vi "Write GPIO Bank.vi"(0 "fpga interface in":refnum<k20>, 5 "gpio bank select":T1, 7 "gpio bank output":T2, 9 "gpio bank output enable":T2={"GPIO 0"=TRUE, "GPIO 1"=TRUE, "GPIO 2"=TRUE, "GPIO 3"=TRUE, "GPIO 4"=TRUE, "GPIO 5"=TRUE, "GPIO 6"=TRUE, "GPIO 7"=TRUE, "GPIO 8"=TRUE, "GPIO 9"=TRUE, "GPIO 10"=TRUE}, 11 "error in (no error)":errorcluster) -> (4 "fpga interface out":refnum<k20>, 15 "error out":errorcluster)   [LabVIEW 2023, in "GettingStarted_Common_148X_Host.lvlib"]
uses:
  GettingStarted_Common_148X_Host.lvlib
  <instrlib>/FlexRIO/CSI-2/v2/FPGA/Types/GPIO Bank.ctl
  FPGA/Common/Types/SerDes Identifier.ctl
  Types/148x_Common_FPGA_Reference.ctl
  <vilib>/rvi/errors/niLvFpgaAdjustHostInterfaceError.vi
  <vilib>/rvi/interface/nirviReadWriteControl/nirviReadWriteControl.xnode
  FPGA/Common/GettingStarted_Common_148X_FPGA.lvlib
  NiFpgaLv.dll
  <vilib>/rvi/interface/Simulation/niFpgaSimulationCallBeginRW.vi
  <instrlib>/FlexRIO/CSI-2/v2/FPGA/NI CSI-2 API FPGA v2.lvlib
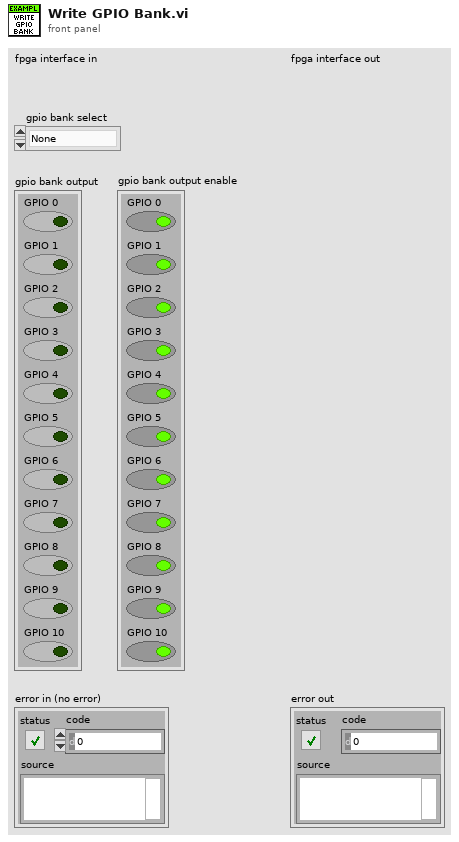
[diagram p1: front panel]
types:
  T1 = typedef "GettingStarted_Common_148X_FPGA.lvlib/SerDes Identifier.ctl" = enum8{"None", "SI 0 Deserializer", "SI 1 Deserializer", "SI 2 Deserializer", "SI 3 Deserializer", "SI 4 Deserializer", "SI 5 Deserializer", "SI 6 Deserializer", "SI 7 Deserializer", "SO 0 Serializer", "SO 1 Serializer", "SO 2 Serializer", "SO 3 Serializer", "SO 4 Serializer", "SO 5 Serializer", "SO 6 Serializer", "SO 7 Serializer", "SI 0 SI 1 Deserializer", "SI 2 SI 3 Deserializer", "SI 4 SI 5 Deserializer", "SI 6 SI 7 Deserializer"}
  T2 = typedef "NI CSI-2 API FPGA v2.lvlib/GPIO Bank.ctl" = cluster{"GPIO 0":bool, "GPIO 1":bool, "GPIO 2":bool, "GPIO 3":bool, "GPIO 4":bool, "GPIO 5":bool, "GPIO 6":bool, "GPIO 7":bool, "GPIO 8":bool, "GPIO 9":bool, "GPIO 10":bool}
  T3 = typedef "GettingStarted_Common_148X_Host.lvlib/148x_Common_FPGA_Reference.ctl" = refnum<k20>
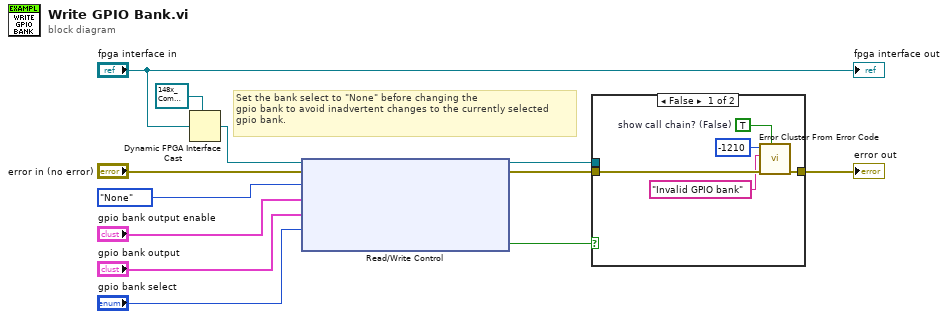
[diagram p0: block diagram]
diagram:
  # "Set the bank select to \"None\" before changing the \ngpio bank to avoid inadvertent changes to the currently selected\ngpio bank."
  n1 = Dynamic FPGA Interface Cast(Session In=T3 refnum ("FPGA VI Reference Out"), Type="fpga interface in") -> (Session Out=w11:T3)
  n2 = xnode "Read/Write Control"("FPGA VI Reference In"=w11, "error in"="error in (no error)", "gpio bank output select"=SerDes_Identifier."None", "gpio bank output enable"="gpio bank output enable", "gpio bank output"="gpio bank output", "gpio bank output select"="gpio bank select") -> ("FPGA VI Reference Out"=w7:T3, "error out"=w8:errorcluster, "serdes gpio bank output select valid"=w3:bool)
  n3 = case shown="False" w3 {
    tunnel: w8 -> [w17 w18]
    tunnel: [w16 w18] -> w6
    tunnel: w7 -> [_ _]
    frame False {
      w13 = TRUE  # show call chain? (False)
      n4 = call <vilib>:"Error Cluster From Error Code.vi"("show call chain? (False)"=w13, "error in (no error)"=w17, "error message (\"\")"="Invalid GPIO bank" ("error message (\"\")"), "error code (0)"=-1210) -> ("error out"=w16:errorcluster)  [unwired: 5 in]
    }
    frame True {
    }
  }
  "error out" <- w6
  "fpga interface out" <- "fpga interface in"
